vi "Traffic Light.vi"() -> ()   [LabVIEW 2014]
panel:
  out "Green":bool
  out "Yellow":bool
  out "Red":bool
  in  "Stop Button":bool
  out "TIMER":dbl(knob) scale=0.0..10.0
  # "TRAFFIC LIGHT"
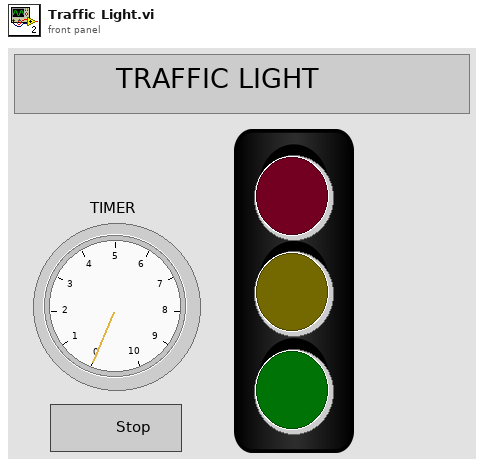
[diagram p1: front panel]
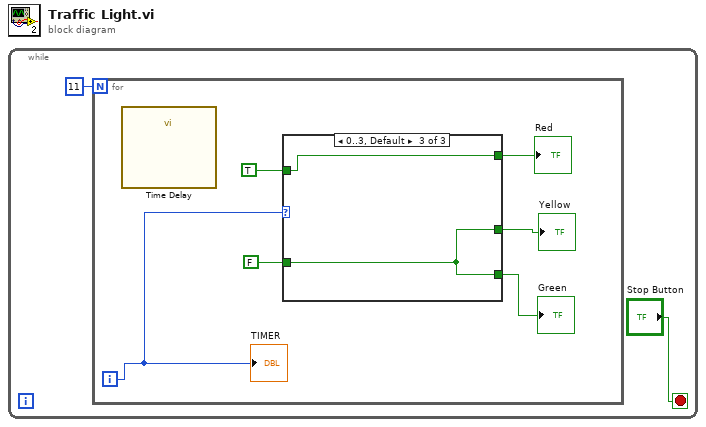
[diagram p0: block diagram]
diagram:
  n1 = while {
    stop <- "Stop Button" stop-if-true
    n2 = for {
      N: 11 -> [_]
      i -> [w8]
      n3 = call "Time Delay"() -> ()  [unwired: 11 in, 1 out]
      n4 = case shown="0..3, Default" w8 {
        tunnel: FALSE -> [w9 w11 w14]
        tunnel: TRUE -> [w10 w12 w13]
        tunnel: [w10 w11 w14] -> w5
        tunnel: [w9 w12 w14] -> w4
        tunnel: [w9 w11 w13] -> w3
        frame 4, 5 {
        }
        frame 6.. {
        }
        frame 0..3, Default {
        }
      }
      "Green" <- w4
      "Yellow" <- w5
      "Red" <- w3
      "TIMER" <- w8
    }
  }
